vi "打码工位查验.vi"(11 "二维码":string) -> (1 "Rows Fetched":i32, 3 "可否打码":bool)   [LabVIEW 2014]
panel:
  out "干检OK":i32
  out "氦检OK":i32
  out "查重信息":string[][](array[string])
  out "error out":errorcluster
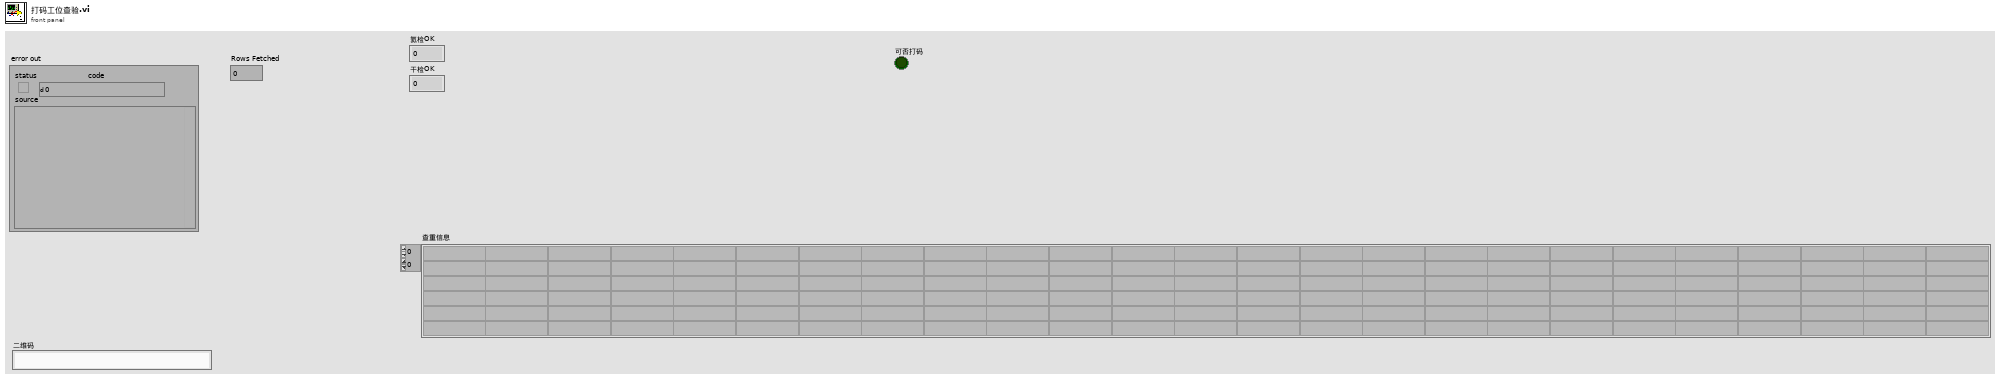
[diagram p1: front panel]
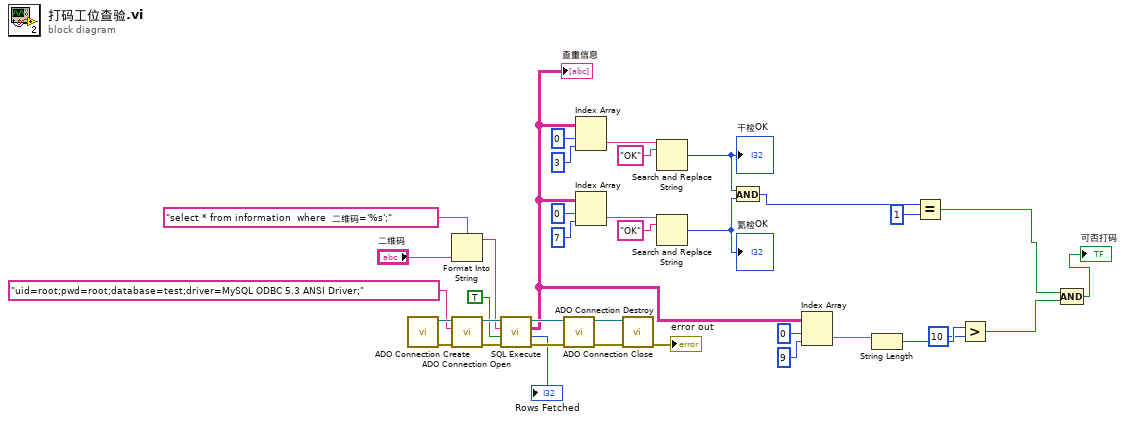
[diagram p0: block diagram]
diagram:
  n1 = call "ADO Connection Create.vi"() -> ("error out"=w35:errorcluster, "ADODB._Connection Out"=w36:refnum<k7>)  [unwired: 10 in]
  n2 = Format Into String(format string="select * from information  where  二维码='%s';" ("Command Text"), "二维码") -> (resulting string=w24:string)  [unwired: 2 in, 1 out]
  n3 = call "ADO Connection Open.vi"("error in (no error)"=w35, "ConnectionString"="uid=root;pwd=root;database=test;driver=MySQL ODBC 5.3 ANSI Driver;", "ADODB._Connection In"=w36) -> ("error out"=w33:errorcluster, "ADODB._Connection Out"=w34:refnum<k7>)  [unwired: 7 in]
  n4 = call "SQL Execute.vi"("error in (no error)"=w33, "Return Data (T)"=TRUE, "Command Text"=w24, "ADODB._Connection In"=w34) -> ("error out"=w31:errorcluster, "Rows Fetched"=→"Rows Fetched":i32, "Data"=w4:string[][], "ADODB._Connection Out"=w32:refnum<k7>)  [unwired: 4 in]
  "查重信息" <- w4
  n5 = call "ADO Connection Close.vi"("error in (no error)"=w31, "ADODB._Connection In"=w32) -> ("error out"=w29:errorcluster, "ADODB._Connection Out"=w30:refnum<k7>)  [unwired: 8 in]
  n6 = Index Array(array=w4, index (row)=0 ("禁用的索引 (行)"), index (col)=3 ("禁用的索引 (列)")) -> (element=w15:string)
  n7 = Index Array(array=w4, index (row)=0 ("禁用的索引 (行)"), index (col)=7 ("禁用的索引 (列)")) -> (element=w18:string)
  n8 = call "ADO Connection Destroy.vi"("error in (no error)"=w29, "ADODB._Connection In"=w30) -> ("error out"=→"error out":errorcluster)  [unwired: 9 in]
  n9 = Search and Replace String(input string=w15, search string="OK" ("搜索字符串")) -> (number of replacements=w13:i32)  [unwired: 6 in, 3 out]
  "干检OK" <- w13
  n10 = Search and Replace String(input string=w18, search string="OK" ("搜索字符串")) -> (number of replacements=w12:i32)  [unwired: 6 in, 3 out]
  "氦检OK" <- w12
  n11 = And(x=w13, y=w12) -> (x .and. y?=w6:i32)
  n12 = Index Array(array=w4, index (row)=0 ("禁用的索引 (行)"), index (col)=9 ("禁用的索引 (列)")) -> (element=w9:string)
  n13 = String Length(string=w9) -> (length=w8:i32)
  n14 = Equal?(x=w6, y=1) -> (x = y?=w3:bool)
  n15 = Greater?(x=w8, y=10) -> (0:w2:bool)
  n16 = Compound Arithmetic op=AND ("复合运算")(w3, w2) -> (→"可否打码":bool)
